vi "Get Channel Groups.vi"(8 "error in (no error)":errorcluster, 11 "File Ref in":refnum<k20>) -> (0 "error out":errorcluster, 2 "Channel Groups":refnum<k20>[](array[refnum]), 3 "File Ref out":refnum<k20>)   [LabVIEW 2019, in "Engine Simulation Toolkit System Explorer.lvlib" / "File Interface.lvlib"]
uses:
  File Interface.lvlib
  <vilib>/Platform/storage/Storage.llb/Get Property (Storage Refnums).vi
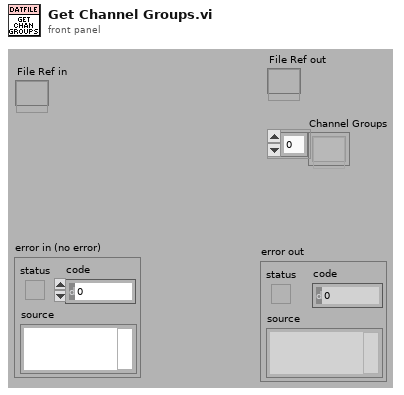
[diagram p1: front panel]
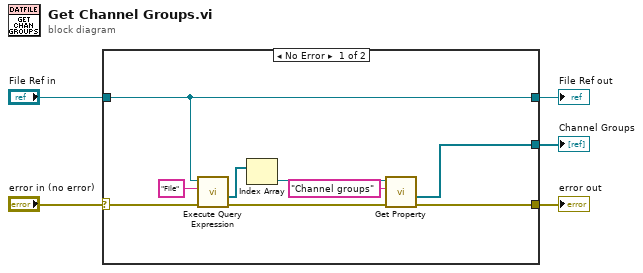
[diagram p0: block diagram]
diagram:
  n1 = case shown="No Error" "error in (no error)" {
    selector: "error in (no error)" -> [w10 w16]
    tunnel: [w6 w16] -> w5
    tunnel: "File Ref in" -> [w8 w15]
    tunnel: [w8 w15] -> w2
    tunnel: [w7 _] -> w1
    frame No Error {
      n2 = call <vilib>:"Execute Query Expression.vi"("error in (no error)"=w10, "object type"="File", "storage refnum"=w8) -> ("error out"=w9:errorcluster, "storage refnums"=w13:refnum<k20>[])  [unwired: 1 in, 2 out]
      n3 = Index Array(array=w13) -> (element=w11:refnum<k20>)  [unwired: 1 in]
      n4 = call-poly <vilib>:"Get Property.vi"("error in (no error)"=w9, "Property name"="Channel groups" ("PropertyName"), "storage refnum"=w11) -> ("error out"=w6:errorcluster, "Value"=w7:refnum<k20>[])  [unwired: 7 out]
    }
    frame Error {
    }
  }
  "File Ref out" <- w2
  "error out" <- w5
  "Channel Groups" <- w1
